vi "MQTT_Publicar_Sensor_Luminosidad.vi"() -> ()   [LabVIEW 2017, in "MQTT_Functions.lvlib"]
doc: "A simple client example that connects to a broker server and publishes messages to a topic.\n\n© 2015 - daq.io, LLC - Peter Adelhardt"
uses:
  MQTT_Functions.lvlib
  Controls/QoS.ctl
  Controls/Retain_Flag.ctl
  Controls/DUP_Flag.ctl
  Controls/Connection_Return_Codes.ctl
  Controls/Connect_Flags.ctl
panel:
  in  "Conexión MQTT":T1={"URL Broker"="broker.mqttdashboard.com", "Puerto de Conexión"=1883}
  out "Gráfico de Medidor":dbl(graph)
  out "Intensidad Baja":bool
  out "Intensidad Media":bool
  out "Intensidad Alta":bool
  out "Medidor":dbl(knob) scale=0.0..100.0
  in  "Tópico":string="sensor/datos/luminosidad"
  out "Mensaje Públicado en Cliente MQTT":string
  in  "Stop Publishing":bool
  out "Message ID (acknowledged)":u16=10
  out "Acknowledged":bool
  in  "Message ID":u16=20
  out "Connection Status":T2=enum."Connection refused: not authorized"
  out "error out":errorcluster
  in  "Client ID":string="LabVIEW_MQTT_Client"
  in  "error in (no error)":errorcluster
  in  "Publish Meta":cluster{"QoS":T3, "Retain":T4, "DUP":T5}
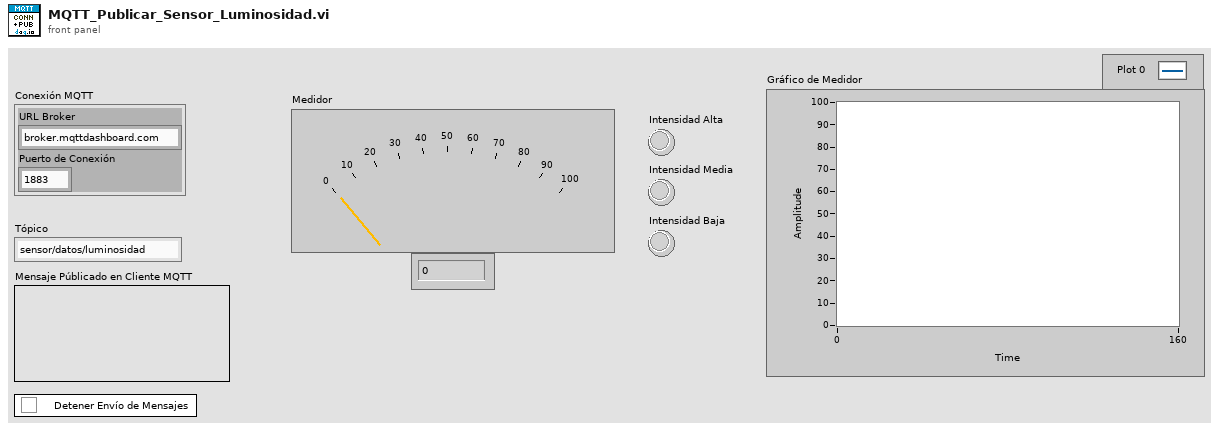
[diagram p1: front panel]
types:
  T1 = cluster{"URL Broker":string, "Puerto de Conexión":i32}
  T2 = typedef "MQTT_Functions.lvlib/Connection_Return_Codes.ctl" = enum16{"Connection accepted", "Connection refused: unacceptable protocol version", "Connection refused: identifier rejected", "Connection refused: Server unavailable", "Connection refused: bad user name or password", "Connection refused: not authorized"}
  T3 = typedef "MQTT_Functions.lvlib/QoS.ctl" = enum8{"At most once", "At least once", "Exactly once", "Reserved"}
  T4 = typedef "MQTT_Functions.lvlib/Retain_Flag.ctl" = bool
  T5 = typedef "MQTT_Functions.lvlib/DUP_Flag.ctl" = bool
  T6 = typedef "MQTT_Functions.lvlib/Connect_Flags.ctl" = cluster{"user name":bool, "password":bool, "will retain":bool, "will flag":bool, "clean session":bool, "reserved":bool, "will QoS":T3}
  T7 = cluster{"QoS":T3, "DUP":T5, "Retain":T4, "Keep Alive (sec)":u16}
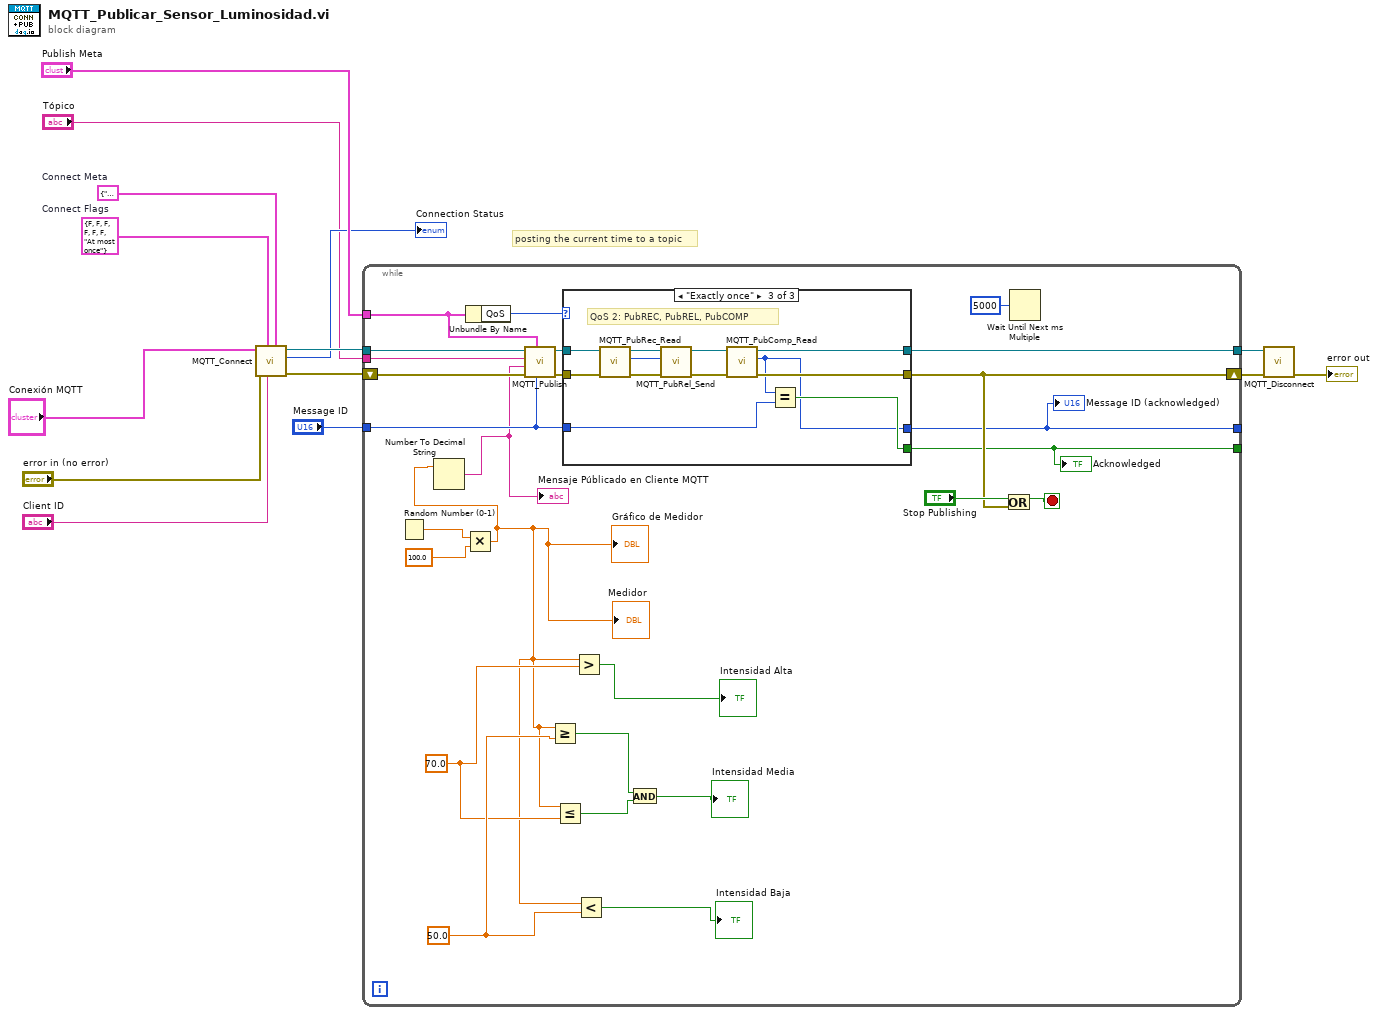
[diagram p0: block diagram]
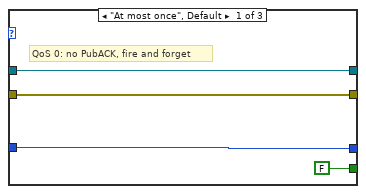
[diagram p2: hidden frame]
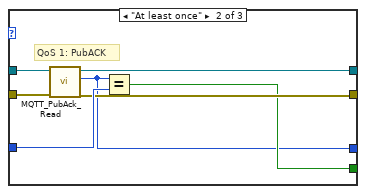
[diagram p3: hidden frame]
diagram:
  w14 = T6 {"user name"=FALSE, "password"=FALSE, "will retain"=FALSE, "will flag"=FALSE, "clean session"=FALSE, "reserved"=FALSE, "will QoS"=enum."At most once"}  # Connect Flags
  w11 = T7 {"QoS"=enum."At most once", "DUP"=FALSE, "Retain"=FALSE, "Keep Alive (sec)"=60}  # Connect Meta
  # "posting the current time to a topic"
  n1 = call "MQTT_Connect.vi"("Connect Meta"=w11, "Client ID"="Client ID", "Connect Flags"=w14, "error in (no error)"="error in (no error)", "MQTT Broker"="Conexión MQTT") -> ("error out"=w3:errorcluster, "Connection Status"=→"Connection Status":T2, "connection ID out"=w5:refnum<k5>)  [unwired: 4 in]
  n2 = while {
    tunnel: "Tópico" -> [w40]
    tunnel: w5 -> [w39]
    tunnel: "Publish Meta" -> [w37]
    tunnel: [w33] -> w7
    tunnel: "Message ID" -> [w32]
    tunnel: [w27] -> _
    tunnel: [w26] -> _
    shift-right: [w29] -> w8
    shift-left: w3 -> [w38]
    stop <- w30 stop-if-true
    w16 = 70.0 ("number (0 to 1)")
    w17 = 50.0 ("number (0 to 1)")
    n3 = Random Number (0-1)() -> (number: 0 to 1=w24:dbl)
    n4 = Multiply(x=w24, y=100.0 ("number (0 to 1)")) -> (x*y=w15:dbl)
    "Medidor" <- w15
    "Gráfico de Medidor" <- w15
    n5 = Number To Decimal String(number=w15) -> (decimal integer string=w25:string)  [unwired: 1 in]
    "Mensaje Públicado en Cliente MQTT" <- w25
    n6 = Unbundle By Name(w37) -> ("QoS"=w36:T3)
    n7 = call "MQTT_Publish.vi"("Message ID"=w32, "Publish Meta"=w37, "error in (no error)"=w38, "Message to be published"=w25, "Topic"=w40, "connection ID"=w39) -> ("error out"=w35:errorcluster, "connection ID out"=w34:refnum<k5>)  [unwired: 4 in]
    n8 = Greater Or Equal?(x=w15, y=w17) -> (x >= y?=w18:bool)
    n9 = Less Or Equal?(x=w15, y=w16) -> (x <= y?=w19:bool)
    n10 = case shown="\"Exactly once\"" w36 {
      tunnel: w35 -> [w43 w50 w62]
      tunnel: w34 -> [w44 w51 w63]
      tunnel: [w43 w48 w55] -> w29
      tunnel: [w44 w47 w56] -> w33
      tunnel: w32 -> [w41 w49 w61]
      tunnel: [FALSE w46 w57] -> w27
      tunnel: [w41 w45 w54] -> w26
      frame "At most once", Default {
        # "QoS 0: no PubACK, fire and forget"
      }
      frame "At least once" {
        # "QoS 1: PubACK"
        n11 = call "MQTT_PubAck_Read.vi"("error in (no error)"=w50, "connection ID"=w51) -> ("error out"=w48:errorcluster, "Message ID"=w45:u16, "connection ID out"=w47:refnum<k5>)  [unwired: 7 in]
        n12 = Equal?(x=w45, y=w49) -> (x = y?=w46:bool)
      }
      frame "Exactly once" {
        # "QoS 2: PubREC, PubREL, PubCOMP"
        n13 = call "MQTT_PubRec_Read.vi"("error in (no error)"=w62, "connection ID"=w63) -> ("error out"=w60:errorcluster, "Message ID"=w58:u16, "connection ID out"=w59:refnum<k5>)  [unwired: 7 in]
        n14 = call "MQTT_PubRel_Send.vi"("error in (no error)"=w60, "Message ID"=w58, "connection ID"=w59) -> ("error out"=w52:errorcluster, "connection ID out"=w53:refnum<k5>)  [unwired: 6 in, 1 out]
        n15 = call "MQTT_PubComp_Read.vi"("error in (no error)"=w52, "connection ID"=w53) -> ("error out"=w55:errorcluster, "Message ID"=w54:u16, "connection ID out"=w56:refnum<k5>)  [unwired: 7 in]
        n16 = Equal?(x=w54, y=w61) -> (x = y?=w57:bool)
      }
    }
    "Message ID (acknowledged)" <- w26
    "Acknowledged" <- w27
    n17 = Greater?(x=w15, y=w16) -> (0:→"Intensidad Alta":bool)
    n18 = Less?(x=w15, y=w17) -> (x < y?=→"Intensidad Baja":bool)
    n19 = And(x=w18, y=w19) -> (x .and. y?=→"Intensidad Media":bool)
    n20 = Or(x="Stop Publishing", y=w29) -> (x .or. y?=w30:bool)
    n21 = Wait Until Next ms Multiple(millisecond multiple=u32 5000) -> ()  [unwired: 1 out]
  }
  n22 = call "MQTT_Disconnect.vi"("error in (no error)"=w8, "connection ID"=w7) -> ("error out"=→"error out":errorcluster)  [unwired: 9 in]
